vi "CameraGetData.vi"(7 "Action":T1, 8 "error in":errorcluster) -> (0 "error out":errorcluster, 2 "occurrence":refnum<k4>)   [LabVIEW 2013]
doc: "Wrapper for an occurence (basically a queue with no data). It has the following actions:\n-Init: generate an occurrence.\n-Get: return a reference to the occurrence.\n-Set: sets the occurrence (notifies all code waiting on the occurence to continue)."
uses:
  OccurrenceAction.ctl
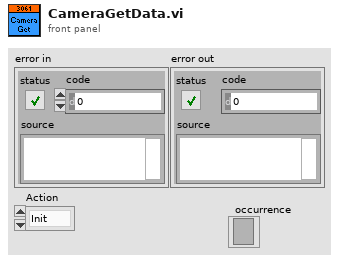
[diagram p1: front panel]
types:
  T1 = typedef "OccurrenceAction.ctl" = enum16{"Init", "Get", "Set"}
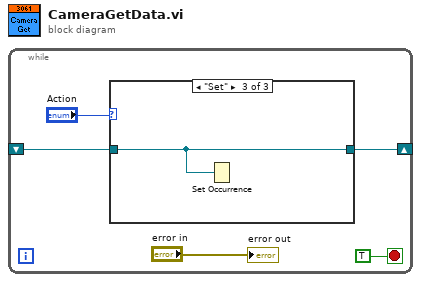
[diagram p0: block diagram]
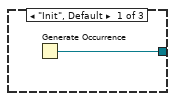
[diagram p2: hidden frame]
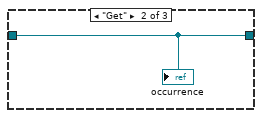
[diagram p3: hidden frame]
diagram:
  n1 = while {
    shift-right: [w4] -> _
    shift-left: _ -> [w3]
    stop <- TRUE stop-if-true
    n2 = case shown="\"Set\"" "Action" {
      tunnel: [w6 w7 w8] -> w4
      tunnel: w3 -> [_ w7 w8]
      frame "Init", Default {
        n3 = Generate Occurrence() -> (w6:refnum<k4>)
      }
      frame "Get" {
        "occurrence" <- w7
      }
      frame "Set" {
        n4 = Set Occurrence(w8) -> ()
      }
    }
    "error out" <- "error in"
  }
